vi "Get Error Message.vi"(8 "error in (no error)":errorcluster, 11 "Connection in":refnum<class "Connection.lvclass">) -> (0 "error out":errorcluster, 2 "error message":string, 3 "Connection out":refnum<class "Connection.lvclass">)   [LabVIEW 2011, in "SQLite.lvlib" / "Connection.lvclass"]
uses:
  Connection.lvclass
  Connection.lvclass/Connection.ctl
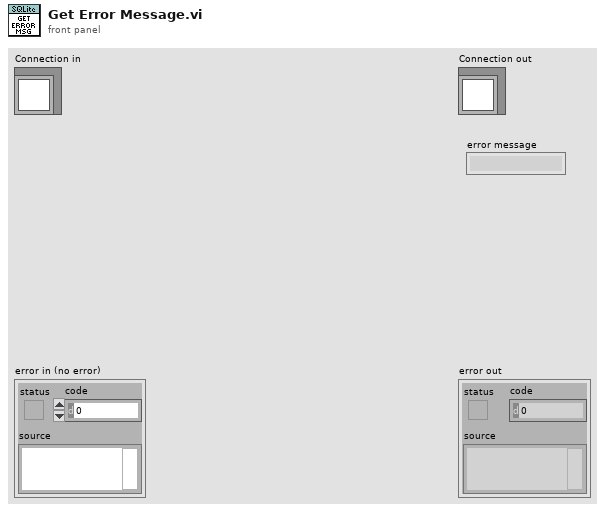
[diagram p1: front panel]
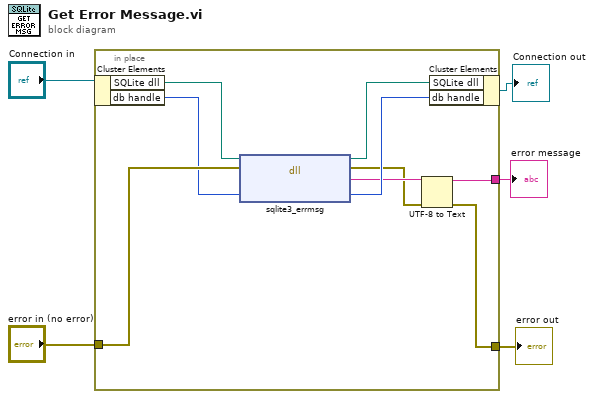
[diagram p0: block diagram]
diagram:
  n1 = in-place {
    in-place-border: "error in (no error)" -> [w14]
    in-place-border: [w6] -> w4
    in-place-border: [w8] -> w3
    n2 = in-place-cluster #1("Connection in") -> ("SQLite dll"=w13:path, "db handle"=w11:u64)
    n3 = dll-call lib="C:/LabVIEW_JDP/Support/SQLite/SQL Connection/sqlite3.dll" fn="sqlite3_errmsg"(path in=w13, error in=w14, "db handle"=w11) -> (path out=w12:path, error out=w7:errorcluster, "error message"=w9:string, "db handle"=w10:u64)  [unwired: 1 in]
    n4 = UTF-8 to Text(8:w7, 11:w9) -> (0:w6:errorcluster, 3:w8:string)
    n5 = in-place-cluster #1("SQLite dll"=w12, "db handle"=w10) -> (→"Connection out":refnum<class "Connection.lvclass">)
  }
  "error out" <- w4
  "error message" <- w3
